vi "PXI-4130 Initialization - Add DCPower Channel.vi"(8 "error in (no error)":errorcluster, 9 "Channel #":i32, 10 "Channel Name":string, 11 "Device Item Ref In":T1 format="%.0x") -> (0 "error out":errorcluster, 3 "Device Item Ref Out":T1 format="%.0x")   [LabVIEW 2009, in "PXI-4130 Custom Device.lvlib"]
uses:
  PXI-4130 Custom Device.lvlib
  <vilib>/NI VeriStand/Custom Device API/Custom Device Item Ref.ctl
  <vilib>/NI VeriStand/Custom Device API/Custom Device Channel Type.ctl
  <vilib>/NI VeriStand/Custom Device API/Custom Device Channel.ctl
  Channel Type.ctl
  Channel Sense.ctl
  PXI-4130 Global Variable.vi
  <vilib>/NI VeriStand/Custom Device API/Set Item Property (I32).vi
  <vilib>/NI VeriStand/Custom Device API/Custom Device API.lvlib
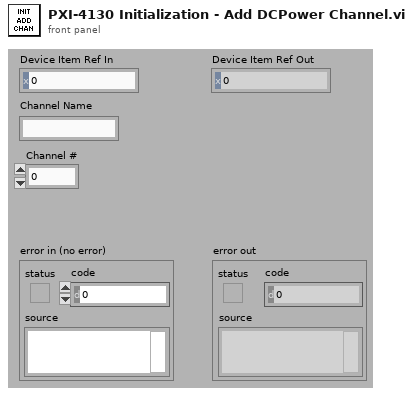
[diagram p1: front panel]
types:
  T1 = typedef "Custom Device API.lvlib/Custom Device Item Ref.ctl" = u64
  T2 = typedef "PXI-4130 Custom Device.lvlib/Channel Sense.ctl" = i32
  T3 = typedef "PXI-4130 Custom Device.lvlib/Channel Type.ctl" = i32
  T4 = typedef "Custom Device API.lvlib/Custom Device Channel Type.ctl" = enum16{"Input", "Output"}
  T5 = typedef "Custom Device API.lvlib/Custom Device Channel.ctl" = cluster{"Type":T4, "Units":string, "Default Value":dbl, "Faultable":bool, "Scalable":bool}
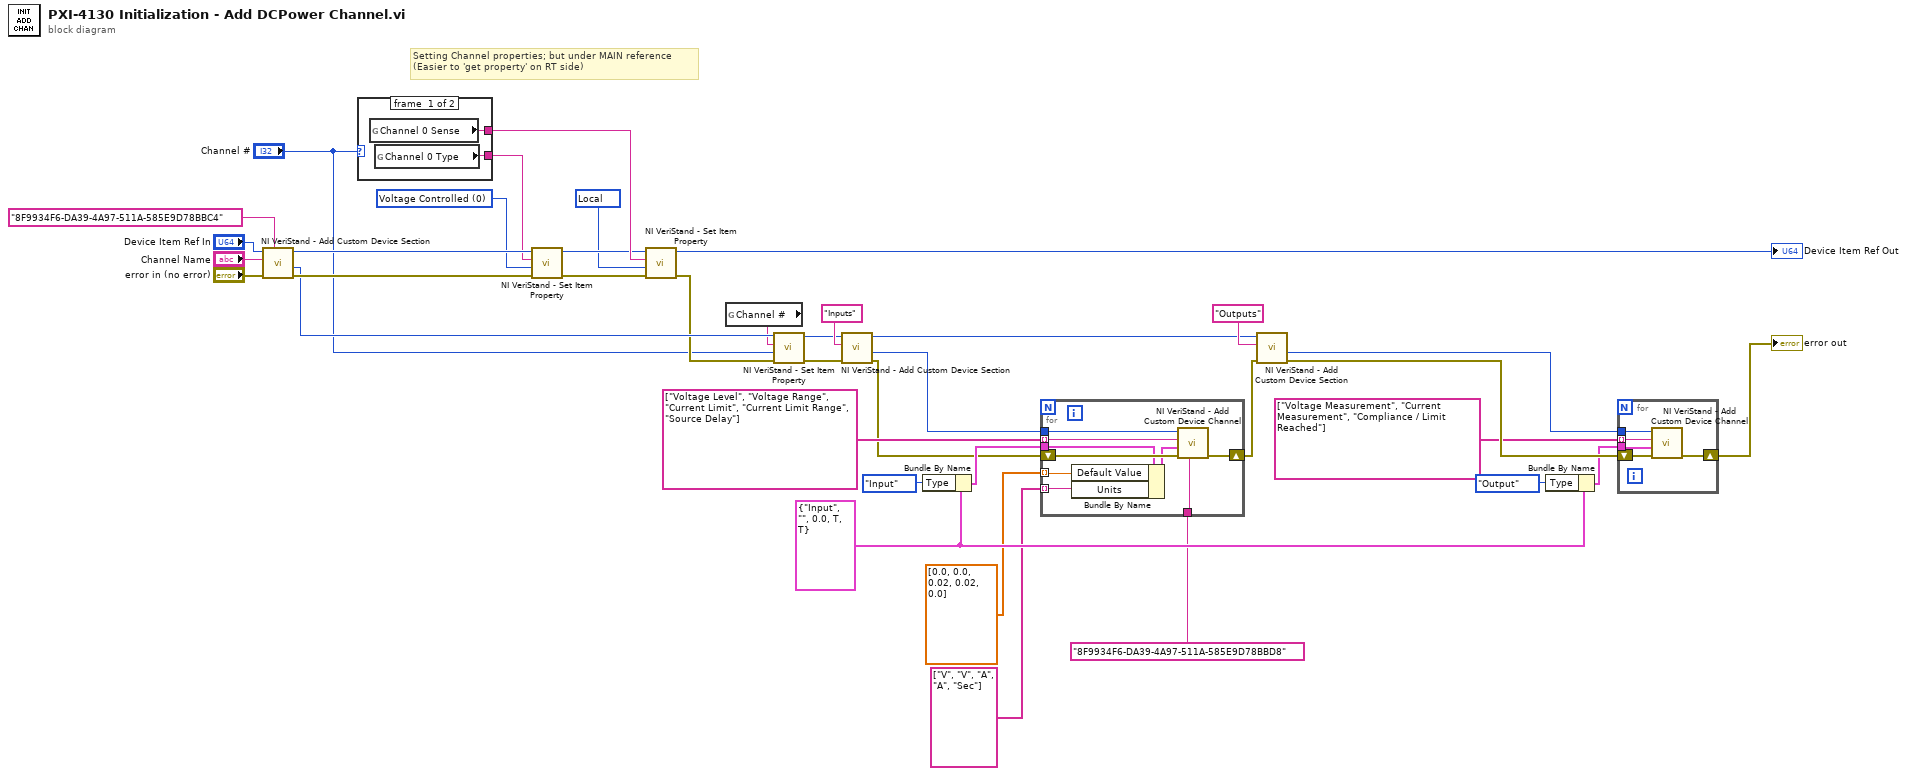
[diagram p0: block diagram]
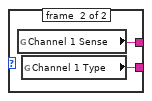
[diagram p2: hidden frame]
diagram:
  w4 = T2 1008 items=["Local"=1008, "Remote"=1009] ("Channel Sense")
  w15 = T3 0 items=["Voltage Controlled", "Current Controlled"] ("Channel Type")
  w22 = T5 {"Type"=enum."Input", "Units"="", "Default Value"=0.0, "Faultable"=TRUE, "Scalable"=TRUE} ("Channel")
  # "Setting Channel properties; but under MAIN reference\n(Easier to 'get property' on RT side)"
  n1 = call <vilib>:"NI VeriStand - Add Custom Device Section.vi"("GUID (Default Section)"="8F9934F6-DA39-4A97-511A-585E9D78BBC4", "error in (no error)"="error in (no error)", "Section Name"="Channel Name", "Parent Ref in"="Device Item Ref In") -> ("error out"=w16:errorcluster, "Section Ptr"=w9:T1, "Parent Ref out"=w20:T1)  [unwired: 5 in]
  n2 = case shown="1" "Channel #" {
    tunnel: [w39 w41] -> w19
    tunnel: [w38 w40] -> w14
    frame #0 {
      n3 = global read "PXI-4130 Global Variable.vi" "Channel 0 Sense"() -> (w38:string)
      n4 = global read "PXI-4130 Global Variable.vi" "Channel 0 Type"() -> (w39:string)
    }
    frame #1 {
      n5 = global read "PXI-4130 Global Variable.vi" "Channel 1 Sense"() -> (w40:string)
      n6 = global read "PXI-4130 Global Variable.vi" "Channel 1 Type"() -> (w41:string)
    }
  }
  n7 = call-poly <vilib>:"NI VeriStand - Set Item Property.vi"("error in (no error)"=w16, "Value"=w15, "Property Name"=w19, "Item Ref in"=w20) -> ("error out"=w8:errorcluster, "Item Ref out"=w13:T1)  [unwired: 5 in, 1 out]
  n8 = call-poly <vilib>:"NI VeriStand - Set Item Property.vi"("Value"=w4, "Property Name"=w14, "Item Ref in"=w13) -> ("Item Ref out"=→"Device Item Ref Out":T1)  [unwired: 6 in, 2 out]
  n9 = global read "PXI-4130 Global Variable.vi" "Channel #"() -> (w6:string)
  n10 = call-poly <vilib>:"NI VeriStand - Set Item Property.vi"("error in (no error)"=w8, "Value"="Channel #", "Property Name"=w6, "Item Ref in"=w9) -> ("error out"=w7:errorcluster, "Item Ref out"=w10:T1)  [unwired: 5 in, 1 out]
  n11 = call <vilib>:"NI VeriStand - Add Custom Device Section.vi"("error in (no error)"=w7, "Section Name"="Inputs", "Parent Ref in"=w10) -> ("error out"=w33:errorcluster, "Section Ptr"=w34:T1, "Parent Ref out"=w18:T1)  [unwired: 6 in]
  n12 = Bundle By Name(cluster=w22, "Type"=Custom_Device_Channel_Type."Input") -> (w35:T5)
  n13 = for {
    tunnel: w34 -> [w50]
    tunnel: string[] ["Voltage Level", "Voltage Range", "Current Limit", "Current Limit Range", "Source Delay"] -> [w48] mode=indexing
    tunnel: w35 -> [w45]
    shift-right: [w47] -> w23
    shift-left: w33 -> [w49]
    tunnel: "8F9934F6-DA39-4A97-511A-585E9D78BBD8" ("Section Name") -> [w46]
    tunnel: dbl[] [0.0, 0.0, 0.02, 0.02, 0.0] -> [w43] mode=indexing
    tunnel: string[] ["V", "V", "A", "A", "Sec"] -> [w42] mode=indexing
    n14 = Bundle By Name(cluster=w45, "Default Value"=w43, "Units"=w42) -> (w44:T5)
    n15 = call <vilib>:"NI VeriStand - Add Custom Device Channel.vi"("GUID (Default Channel)"=w46, "error in (no error)"=w49, "Channel"=w44, "Channel Name"=w48, "Parent Ref in"=w50) -> ("error out"=w47:errorcluster)  [unwired: 4 in, 2 out]
  }
  n16 = call <vilib>:"NI VeriStand - Add Custom Device Section.vi"("error in (no error)"=w23, "Section Name"="Outputs", "Parent Ref in"=w18) -> ("error out"=w31:errorcluster, "Section Ptr"=w30:T1)  [unwired: 6 in, 1 out]
  n17 = Bundle By Name(cluster=w22, "Type"=Custom_Device_Channel_Type."Output") -> (w29:T5)
  n18 = for {
    tunnel: w30 -> [w55]
    tunnel: string[] ["Voltage Measurement", "Current Measurement", "Compliance / Limit Reached"] -> [w53] mode=indexing
    tunnel: w29 -> [w52]
    shift-right: [w51] -> w21
    shift-left: w31 -> [w54]
    n19 = call <vilib>:"NI VeriStand - Add Custom Device Channel.vi"("error in (no error)"=w54, "Channel"=w52, "Channel Name"=w53, "Parent Ref in"=w55) -> ("error out"=w51:errorcluster)  [unwired: 5 in, 2 out]
  }
  "error out" <- w21
